vi "Create Group Indexing.vi"(8 "error in (no error)":errorcluster, 10 "Channels":string[](array[string]), 11 "DAQmxDI in":refnum<class "DAQmxDI.lvclass">) -> (0 "error out":errorcluster, 3 "DAQmxDI out":refnum<class "DAQmxDI.lvclass">)   [LabVIEW 2020, in "VolatusDAQ.lvlib" / "DAQmxDI.lvclass"]
uses:
  DAQmxDI.lvclass
  DAQmxDI.lvclass/DAQmxDI.ctl
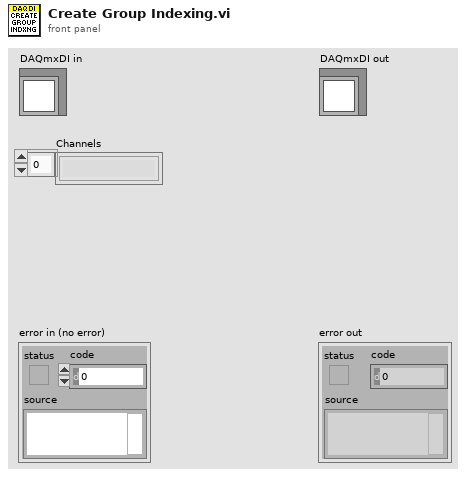
[diagram p1: front panel]
types:
  T1 = typedef "VolatusDAQ.lvlib/DAQmxDI.lvclass/Port Info.ctl" = cluster{"Module Alias":string, "Number":i32, "# Lines":i32, "Lines":map{i32, string}, "Channel Indices":i32[]}
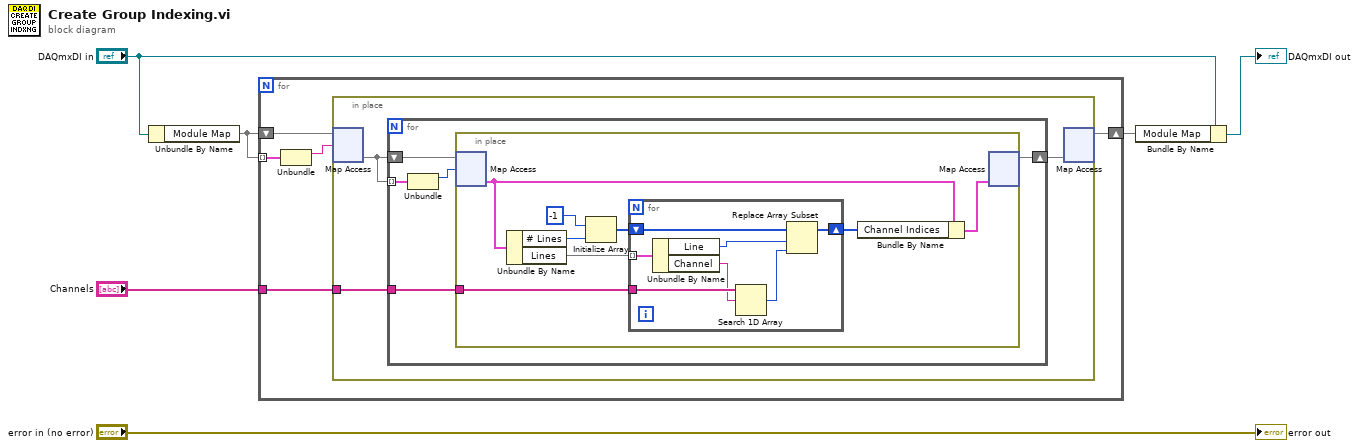
[diagram p0: block diagram]
diagram:
  n1 = Unbundle By Name("DAQmxDI in") -> ("Module Map"=w4:map{string, map{i32, T1}})
  n2 = for {
    shift-right: [w8] -> w2
    shift-left: w4 -> [w10]
    tunnel: w4 -> [w11] mode=indexing
    tunnel: "Channels" -> [w7]
    n3 = Unbundle(w11) -> ("Module Alias"=w9:string)  [unwired: 1 out]
    n4 = in-place {
      in-place-border: w7 -> [w12]
      n5 = in-place-map #1(w10, w9) -> (w14:map{i32, T1})  [unwired: 1 in, 1 out]
      n6 = for {
        shift-right: [w16] -> w13
        shift-left: w14 -> [w18]
        tunnel: w14 -> [w19] mode=indexing
        tunnel: w12 -> [w15]
        n7 = Unbundle(w19) -> ("Port"=w17:i32)  [unwired: 1 out]
        n8 = in-place {
          in-place-border: w15 -> [w25]
          n9 = in-place-map #2(w18, w17) -> (w22:T1)  [unwired: 1 in, 1 out]
          n10 = Unbundle By Name(w22) -> ("# Lines"=w27:i32, "Lines"=w23:map{i32, string})
          n11 = Initialize Array(-1 ("element"), w27) -> (w24:i32[])
          n12 = for {
            tunnel: w25 -> [w33]
            shift-right: [w28] -> w21
            shift-left: w24 -> [w31]
            tunnel: w23 -> [w34] mode=indexing
            n13 = Unbundle By Name(w34) -> ("Line"=w30:i32, "Channel"=w32:string)
            n14 = Search 1D Array(1D array=w33, element=w32) -> (index of element=w29:i32)  [unwired: 1 in]
            n15 = Replace Array Subset(array=w31, new element=w29, index=w30) -> (w28:i32[])
          }
          n16 = Bundle By Name(cluster=w22, "Channel Indices"=w21) -> (w20:T1)
          n17 = in-place-map #2(w20) -> (w16:map{i32, T1})  [unwired: 1 in, 2 out]
        }
      }
      n18 = in-place-map #1(w13) -> (w8:map{string, map{i32, T1}})  [unwired: 1 in, 2 out]
    }
  }
  n19 = Bundle By Name(cluster="DAQmxDI in", "Module Map"=w2) -> (→"DAQmxDI out":refnum<class "DAQmxDI.lvclass">)
  "error out" <- "error in (no error)"
